vi "CSVFormat_Rx.vi"(10 "TV Parameters(DataType)":T2 {"Standard" items=["80211A/G/J/P OFDM", "80211B/G DSSS", "80211G DSSSOFDM", "80211N MIMOOFDM", "80211AC MIMOOFDM"]; "OFDM Data Rate (Mbps)" items=["6", "9", "12", "18", "24", "36", "48", "54"]; "80211n PLCP Frame Format" items=["Mixed Format", "Greenfield Format"]; "FEC Coding Type" items=["BCC", "LDPC"]; "DSSS Data Rate (Mbps)" items=["1", "2", "5.5 CCK", "5.5 PBCC", "11 CCK", "11 PBCC", "22", "33"]}, 11 "WLAN RX Result":T1) -> (3 "Rx Row":string[](array[string]))   [LabVIEW 2014]
uses:
  TV/RW/Includes/WLAN - TV - RW - INC - TV_DataType_Cluster.ctl
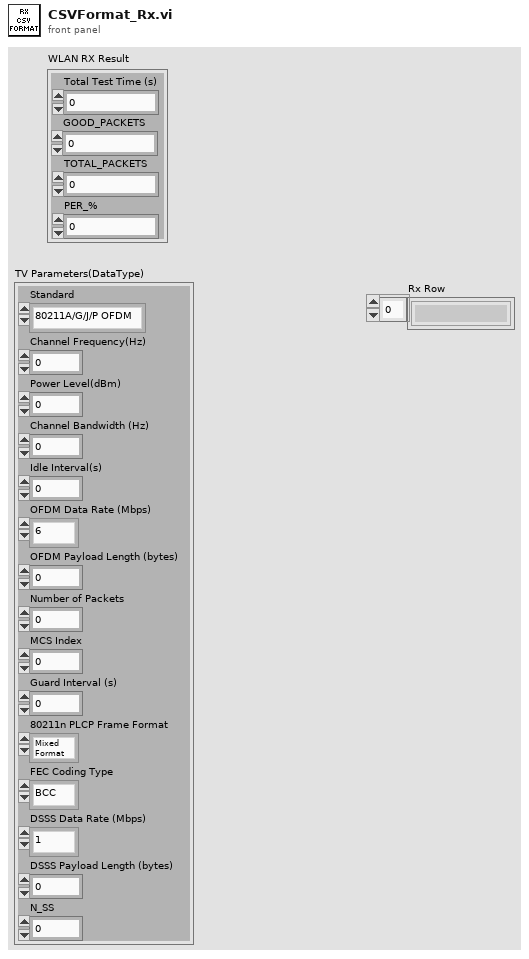
[diagram p1: front panel]
types:
  T1 = cluster{"Total Test Time (s)":dbl, "GOOD_PACKETS":i32, "TOTAL_PACKETS":i32, "PER_%":dbl}
  T2 = typedef "WLAN - TV - RW - INC - TV_DataType_Cluster.ctl" = cluster{"Standard":i32, "Channel Frequency(Hz)":dbl, "Power Level(dBm)":dbl, "Channel Bandwidth (Hz)":dbl, "Idle Interval(s)":dbl, "OFDM Data Rate (Mbps)":i32, "OFDM Payload Length (bytes)":i32, "Number of Packets":i32, "MCS Index":i32, "Guard Interval (s)":dbl, "80211n PLCP Frame Format":i32, "FEC Coding Type":i32, "DSSS Data Rate (Mbps)":i32, "DSSS Payload Length (bytes)":i32, "N_SS":i32}
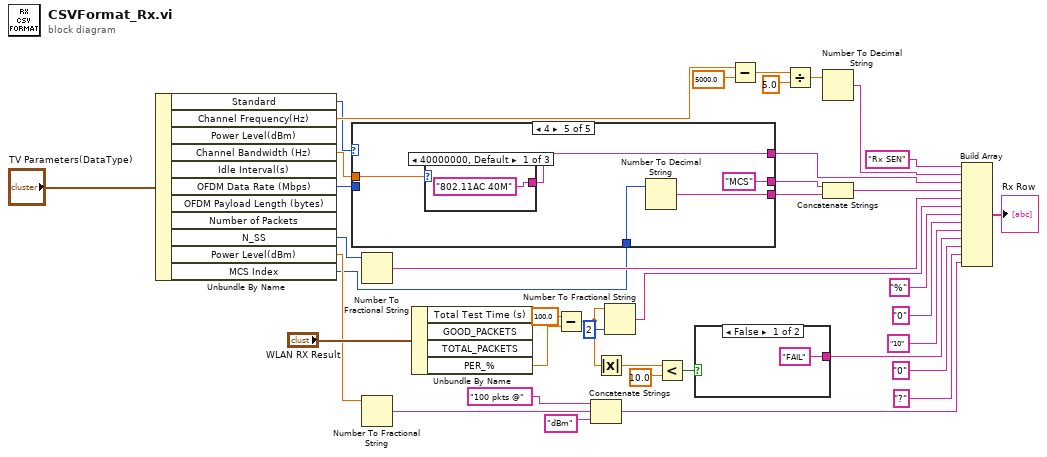
[diagram p0: block diagram]
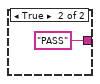
[diagram p2: hidden frame]
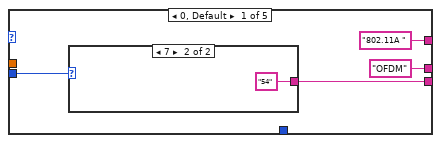
[diagram p3: hidden frame]
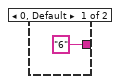
[diagram p4: hidden frame]
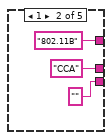
[diagram p5: hidden frame]
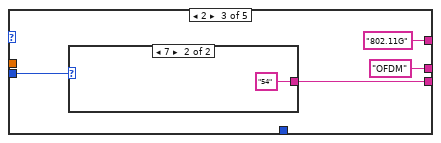
[diagram p6: hidden frame]
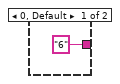
[diagram p7: hidden frame]
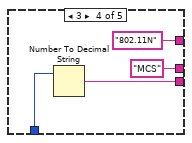
[diagram p8: hidden frame]
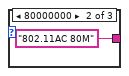
[diagram p9: hidden frame]
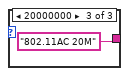
[diagram p10: hidden frame]
diagram:
  n1 = Unbundle By Name("TV Parameters(DataType)") -> ("Standard"=w17:i32, "Channel Frequency(Hz)"=w23:dbl, "Channel Bandwidth (Hz)"=w1:dbl, "OFDM Data Rate (Mbps)"=w14:i32, "N_SS"=w20:i32, "Power Level(dBm)"=w8:dbl, "MCS Index"=w3:i32)  [unwired: 4 out]
  n2 = case shown="4" w17 {
    tunnel: ["802.11A " "802.11B" "802.11G" "802.11N" w59] -> w18
    tunnel: ["OFDM" "CCA" "OFDM" "MCS" "MCS"] -> w19
    tunnel: w14 -> [w41 _ w49 _ _]
    tunnel: [w40 "" w50 w56 w62] -> w13
    tunnel: w3 -> [_ _ _ w55 w61]
    tunnel: w1 -> [_ _ _ _ w60]
    frame 0, Default {
      n3 = case shown="7" w41 {
        tunnel: ["6" "54"] -> w40
        frame 0, Default {
        }
        frame 7 {
        }
      }
    }
    frame 1 {
    }
    frame 2 {
      n4 = case shown="7" w49 {
        tunnel: ["6" "54"] -> w50
        frame 0, Default {
        }
        frame 7 {
        }
      }
    }
    frame 3 {
      n5 = Number To Decimal String(number=w55) -> (decimal integer string=w56:string)  [unwired: 1 in]
    }
    frame 4 {
      n6 = case shown="40000000, Default" w60 {
        tunnel: ["802.11AC 40M" "802.11AC 80M" "802.11AC 20M"] -> w59
        frame 40000000, Default {
        }
        frame 80000000 {
        }
        frame 20000000 {
        }
      }
      n7 = Number To Decimal String(number=w61) -> (decimal integer string=w62:string)  [unwired: 1 in]
    }
  }
  n8 = Number To Fractional String(number=w20) -> (F-format string=w21:string)  [unwired: 3 in]
  n9 = Number To Fractional String(number=w8) -> (F-format string=w9:string)  [unwired: 3 in]
  n10 = Unbundle By Name("WLAN RX Result") -> ("PER_%"=w5:dbl)  [unwired: 3 out]
  n11 = Subtract(x=100.0, y=w5) -> (x-y=w4:dbl)
  n12 = Concatenate Strings("100 pkts @", w9, "dBm" ("string")) -> (w39:string)
  n13 = Absolute Value(x=w4) -> (abs(x)=w34:dbl)
  n14 = Number To Fractional String(number=w4, precision (6)=i16 2) -> (F-format string=w22:string)  [unwired: 2 in]
  n15 = Less?(x=w34, y=10.0) -> (x < y?=w36:bool)
  n16 = case shown="False" w36 {
    tunnel: ["FAIL" ("string") "PASS" ("string")] -> w10
    frame False {
    }
    frame True {
    }
  }
  n17 = Subtract(x=w23, y=5000.0) -> (x-y=w25:dbl)
  n18 = Divide(x=w25, y=5.0) -> (x/y=w27:dbl)
  n19 = Number To Decimal String(number=w27) -> (decimal integer string=w28:string)  [unwired: 1 in]
  n20 = Concatenate Strings(w19, w13) -> (w31:string)
  n21 = Build Array("Rx SEN", w28, w18, w31, w21, w22, "%" ("element"), "0" ("element"), "10" ("element"), w10, "0" ("element"), "?" ("element"), w39) -> (→"Rx Row":string[])
